vi "Read Axis Labels.vi"(8 "error in (no error)":errorcluster, 11 "MAS in":refnum<class "MAS.lvclass">) -> (0 "error out":errorcluster, 2 "Axis Labels":string[](array[string]), 3 "MAS out":refnum<class "MAS.lvclass">)   [LabVIEW 2022 SP3, in "MAS.lvclass"]
uses:
  MAS.lvclass
  MAS.lvclass/MAS.ctl
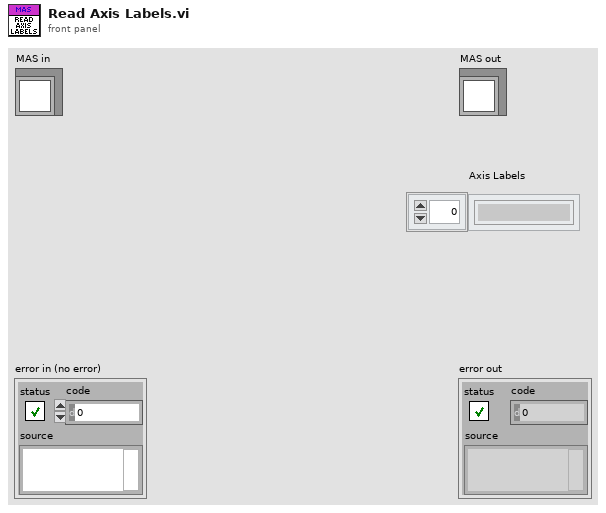
[diagram p1: front panel]
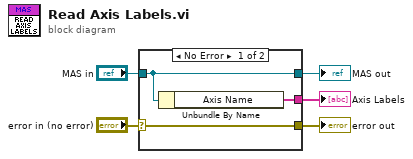
[diagram p0: block diagram]
diagram:
  n1 = case shown="No Error" "error in (no error)" {
    selector: "error in (no error)" -> [w8 w10]
    tunnel: [w8 w10] -> w4
    tunnel: [w7 w9] -> w2
    tunnel: "MAS in" -> [w7 w9]
    tunnel: [w6 _] -> w1
    frame No Error {
      n2 = Unbundle By Name(w7) -> ("Axis Name"=w6:string[])
    }
    frame Error {
    }
  }
  "error out" <- w4
  "MAS out" <- w2
  "Axis Labels" <- w1
